vi "整体初始化.vi"(8 "错误输入（无错误）":errorcluster, 9 "大小":i32, 11 "Scintilla":refnum<k24>) -> (0 "错误输出":errorcluster, 3 "引用输出":refnum<k24>)   [LabVIEW 2020]
uses:
  D:/SuperPython-master/ScintillaNET.dll
  ScintillaNET.dll
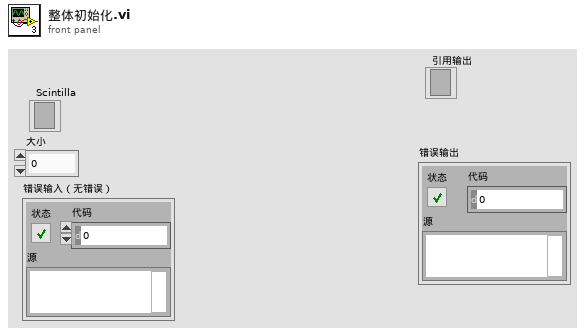
[diagram p1: front panel]
types:
  T1 = cluster{"大小":i32, "粗体":bool, "下划线":bool, "斜体":bool, "背景色":u32, "前景色":u32, "Font":string}
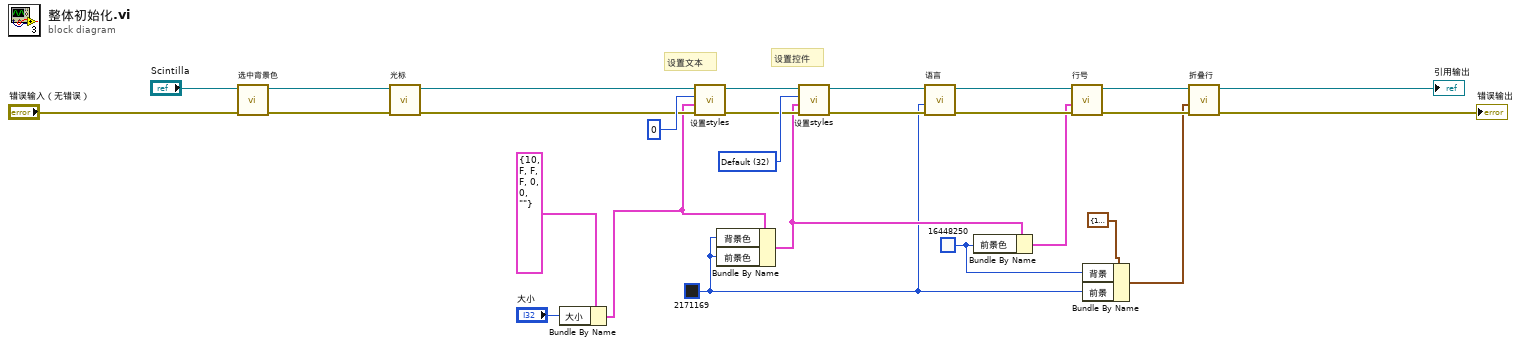
[diagram p0: block diagram]
diagram:
  w10 = u32 16448250 ("前景色")
  w11 = u32 2171169 ("前景色")
  w22 = 32 items=["Default"=32, "LineNumber"=33, "BraceLight"=34, "BraceBad"=35, "IndentGuide"=37, "CallTip"=38, "FoldDisaplayText"=39] ("设置项")
  # "设置控件"
  # "设置文本"
  n1 = call "选中背景色.vi"("错误输入（无错误）"="错误输入（无错误）", "引用"="Scintilla") -> ("错误输出"=w7:errorcluster, "引用输出"=w8:refnum<k24>)  [unwired: 8 in]
  n2 = call "光标.vi"("错误输入"=w7, "引用"=w8) -> ("错误输出"=w5:errorcluster, "引用输出"=w6:refnum<k24>)  [unwired: 8 in]
  n3 = Bundle By Name(cluster=T1 {"大小"=10, "粗体"=FALSE, "下划线"=FALSE, "斜体"=FALSE, "背景色"=0, "前景色"=0, "Font"=""} ("外观属性"), "大小"="大小") -> (w1:T1)
  n4 = call "设置styles.vi"("错误输入（无错误）"=w5, "外观属性"=w1, "设置项"=0, "Scintilla"=w6) -> ("错误输出"=w20:errorcluster, "Scintilla"=w21:refnum<k24>)  [unwired: 6 in]
  n5 = Bundle By Name(cluster=w1, "背景色"=w11, "前景色"=w11) -> (w14:T1)
  n6 = call "设置styles.vi"("错误输入（无错误）"=w20, "外观属性"=w14, "设置项"=w22, "Scintilla"=w21) -> ("错误输出"=w17:errorcluster, "Scintilla"=w18:refnum<k24>)  [unwired: 6 in]
  n7 = call "语言.vi"("错误输入（无错误）"=w17, "背景色"=w11, "Scintilla"=w18) -> ("错误输出"=w15:errorcluster, "Scintilla"=w16:refnum<k24>)  [unwired: 7 in]
  n8 = Bundle By Name(cluster=w14, "前景色"=w10) -> (w13:T1)
  n9 = call "行号.vi"("错误输入（无错误）"=w15, "外观属性"=w13, "Scintilla"=w16) -> ("错误输出"=w23:errorcluster, "引用输出"=w24:refnum<k24>)  [unwired: 7 in]
  n10 = Bundle By Name(cluster=cluster{"背景":u32, "前景":u32} {"背景"=16448250, "前景"=16448250} ("簇"), "背景"=w10, "前景"=w11) -> (w9:cluster{"背景":u32, "前景":u32})
  n11 = call "折叠行.vi"("错误输入（无错误）"=w23, "簇"=w9, "引用"=w24) -> ("错误输出"=→"错误输出":errorcluster, "Scintilla"=→"引用输出":refnum<k24>)  [unwired: 7 in]
